vi "PicoScope4000GetBlock.vi"(0 "error in":errorcluster, 2 "handle in":i16, 3 "Acquisition Settings":T3 {"Down Sample Ratio" min=1 step=1}) -> (4 "overflow":i16, 6 "error out":errorcluster, 7 "handle out":i16, 9 "Buffers (Max or non-aggregated)":T1, 10 "Min Buffers":T2)   [LabVIEW 2009]
doc: "This VI collects a block of data from the oscilloscope. This can be called in a loop in order to continually collect blocks of data. The oscilloscope should first be set up by using PicoScope4000Settings.vi. The VI outputs data arrays in two clusters (max and min). If not using aggregation, 'Min Buffers' is not used."
uses:
  ps4000.dll
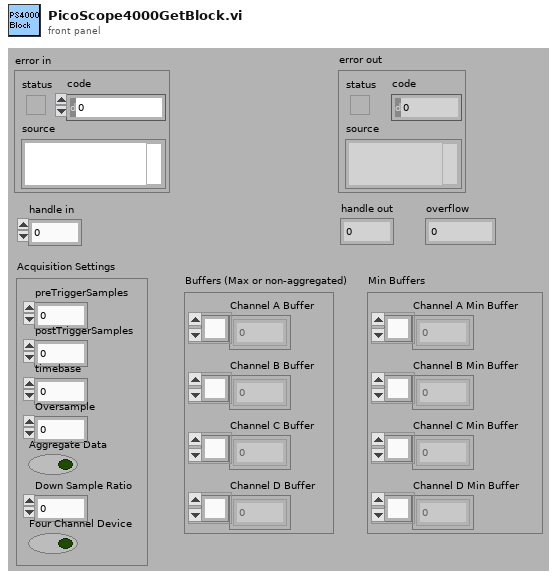
[diagram p1: front panel]
types:
  T1 = cluster{"Channel D Buffer":i16[], "Channel C Buffer":i16[], "Channel B Buffer":i16[], "Channel A Buffer":i16[]}
  T2 = cluster{"Channel A Min Buffer":i16[], "Channel B Min Buffer":i16[], "Channel C Min Buffer":i16[], "Channel D Min Buffer":i16[]}
  T3 = cluster{"preTriggerSamples":i32, "postTriggerSamples":i32, "timebase":u32, "Aggregate Data":bool, "Down Sample Ratio":u32, "Four Channel Device":bool, "Oversample":i16}
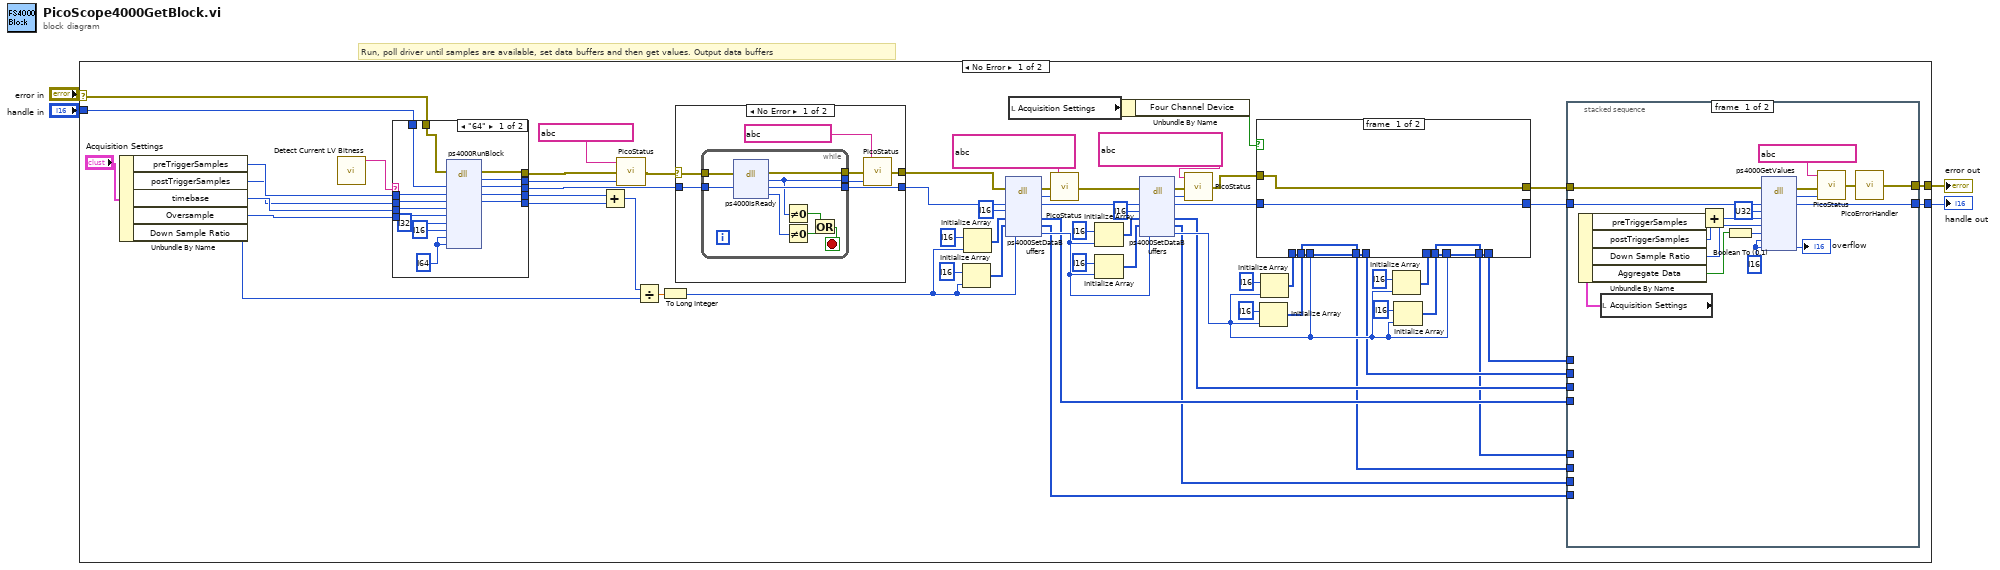
[diagram p0: block diagram]
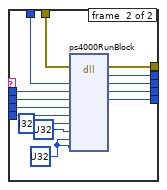
[diagram p2: hidden frame]
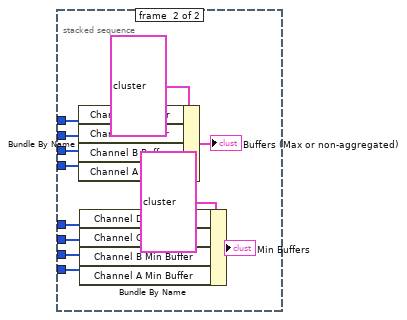
[diagram p3: hidden frame]
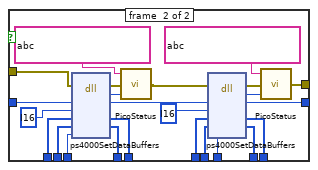
[diagram p5: hidden frame]
diagram:
  # "Run, poll driver until samples are available, set data buffers and then get values. Output data buffers"
  n1 = case shown="No Error" "error in" {
    selector: "error in" -> [w33 w177]
    tunnel: [w34 w177] -> w3
    tunnel: "handle in" -> [w32 w176]
    tunnel: [w31 w176] -> w1
    frame #0 {
      n2 = Unbundle By Name("Acquisition Settings") -> ("preTriggerSamples"=w50:i32, "postTriggerSamples"=w49:i32, "timebase"=w51:u32, "Oversample"=w6:i16, "Down Sample Ratio"=w7:u32)
      n3 = call "Detect Current LV Bitness.vi"() -> ("bitness"=w5:string)  [unwired: 11 in]
      n4 = case shown="\"64\"" w5 {
        tunnel: [w72 w97] -> w69
        tunnel: [w71 w96] -> w64
        tunnel: [w70 w95] -> w63
        tunnel: w51 -> [w79 w94]
        tunnel: w50 -> [w81 w93]
        tunnel: w49 -> [w80 w92]
        tunnel: [w73 w91] -> w46
        tunnel: [w74 w90] -> w45
        tunnel: w33 -> [w83 w89]
        tunnel: w32 -> [w82 w88]
        tunnel: w6 -> [w78 w87]
        frame #0 {
          w75 = i64 ? ("lpReady")
          n5 = dll-call lib="ps4000.dll" fn="ps4000RunBlock" ("ps3000.dll:_ps3000_open_unit@0")(error in=w83, "handle"=w82, "preTriggerSamples"=w81, "postTriggerSamples"=w80, "timebase"=w79, "oversample"=w78, "timeindisposed"=i32 ?, "segmentIndex"=i16 ?, "lpReady"=w75, "pParameter"=w75) -> (error out=w74:errorcluster, "PICO_STATUS"=w73:i32, "handle"=w72:i16, "preTriggerSamples"=w71:i32, "postTriggerSamples"=w70:i32)  [unwired: 8 in, 1 out]
        }
        frame #1 {
          w84 = u32 ? ("lpReady")
          n6 = dll-call lib="ps4000.dll" fn="ps4000RunBlock" ("ps3000.dll:_ps3000_open_unit@0")(error in=w89, "handle"=w88, "preTriggerSamples"=w93, "postTriggerSamples"=w92, "timebase"=w94, "oversample"=w87, "timeindisposed"=i32 ?, "segmentIndex"=u32 ?, "lpReady"=w84, "pParameter"=w84) -> (error out=w90:errorcluster, "PICO_STATUS"=w91:i32, "handle"=w97:i16, "preTriggerSamples"=w96:i32, "postTriggerSamples"=w95:i32)  [unwired: 8 in, 1 out]
        }
      }
      n7 = Add(x=w64, y=w63) -> (x+y=w10:i32)
      n8 = call "PicoStatus.vi"("PICO STATUS"=w46, "error in"=w45, "source"=string ?) -> ("error out"=w44:errorcluster)
      n9 = Divide(x=w10, y=w7) -> (x/y=w9:dbl)
      n10 = To Long Integer(number=w9) -> (32bit integer=w8:i32)
      n11 = case shown="No Error" w44 {
        selector: w44 -> [w132 w144]
        tunnel: w69 -> [w134 w145]
        tunnel: [w133 w145] -> w68
        tunnel: [w131 w144] -> w55
        frame #0 {
          n12 = while {
            tunnel: [w143] -> w133
            tunnel: w134 -> [w142]
            tunnel: [w137] -> w129
            tunnel: w132 -> [w136]
            tunnel: [w135] -> w130
            stop <- w141 stop-if-true
            n13 = dll-call lib="ps4000.dll" fn="ps4000IsReady" ("ps3000.dll:_ps3000_open_unit@0")(error in=w136, "handle"=w142) -> (error out=w135:errorcluster, "status"=w137:i32, "handle"=w143:i16, "ready"=w138:i16)  [unwired: 3 in, 1 out]
            n14 = Not Equal To 0?(x=w137) -> (x != 0?=w139:bool)
            n15 = Not Equal To 0?(x=w138) -> (x != 0?=w140:bool)
            n16 = Or(x=w139, y=w140) -> (x .or. y?=w141:bool)
          }
          n17 = call "PicoStatus.vi"("PICO STATUS"=w129, "error in"=w130, "source"=string ?) -> ("error out"=w131:errorcluster)
        }
        frame #1 {
        }
      }
      n18 = Initialize Array(i16 ? ("element"), w8) -> (w29:i16[])
      n19 = Initialize Array(i16 ? ("element"), w8) -> (w62:i16[])
      n20 = dll-call lib="ps4000.dll" fn="ps4000SetDataBuffers" ("ps3000.dll:_ps3000_open_unit@0")(error in=w55, "handle"=w68, "channel"=i16 ?, "bufferMax"=w62, "bufferMin"=w29, "bufferLth"=w8) -> (error out=w42:errorcluster, "PICO_STATUS"=w43:i32, "handle"=w67:i16, "bufferMax"=w15:i16[], "bufferMin"=w11:i16[], "bufferLth"=w20:i32)  [unwired: 3 in, 1 out]
      n21 = local read "Acquisition Settings"() -> (w48:T3)
      n22 = call "PicoStatus.vi"("PICO STATUS"=w43, "error in"=w42, "source"=string ?) -> ("error out"=w41:errorcluster)
      n23 = Initialize Array(i16 ? ("element"), w20) -> (w59:i16[])
      n24 = Initialize Array(i16 ? ("element"), w20) -> (w27:i16[])
      n25 = Unbundle By Name(w48) -> ("Four Channel Device"=w47:bool)
      n26 = dll-call lib="ps4000.dll" fn="ps4000SetDataBuffers" ("ps3000.dll:_ps3000_open_unit@0")(error in=w41, "handle"=w67, "channel"=i16 ?, "bufferMax"=w59, "bufferMin"=w27, "bufferLth"=w20) -> (error out=w39:errorcluster, "PICO_STATUS"=w40:i32, "handle"=w66:i16, "bufferMax"=w16:i16[], "bufferMin"=w12:i16[], "bufferLth"=w19:i32)  [unwired: 3 in, 1 out]
      n27 = call "PicoStatus.vi"("PICO STATUS"=w40, "error in"=w39, "source"=string ?) -> ("error out"=w38:errorcluster)
      n28 = Initialize Array(i16 ? ("element"), w19) -> (w24:i16[])
      n29 = Initialize Array(i16 ? ("element"), w19) -> (w58:i16[])
      n30 = Initialize Array(i16 ? ("element"), w19) -> (w57:i16[])
      n31 = Initialize Array(i16 ? ("element"), w19) -> (w21:i16[])
      n32 = case shown="True" w47 {
        tunnel: w66 -> [w149 w175]
        tunnel: [w149 w173] -> w65
        tunnel: w58 -> [w151 w172]
        tunnel: w57 -> [w150 w171]
        tunnel: [w150 w170] -> w18
        tunnel: [w151 w169] -> w17
        tunnel: w38 -> [w148 w166]
        tunnel: [w148 w160] -> w53
        tunnel: w24 -> [w147 w157]
        tunnel: w21 -> [w146 w156]
        tunnel: [w146 w155] -> w14
        tunnel: [w147 w154] -> w13
        tunnel: w19 -> [_ w153]
        tunnel: w19 -> [_ w152]
        frame #0 {
        }
        frame #1 {
          n33 = dll-call lib="ps4000.dll" fn="ps4000SetDataBuffers" ("ps3000.dll:_ps3000_open_unit@0")(error in=w166, "handle"=w175, "channel"=i16 ?, "bufferMax"=w172, "bufferMin"=w157, "bufferLth"=w153) -> (error out=w164:errorcluster, "PICO_STATUS"=w165:i32, "handle"=w174:i16, "bufferMax"=w169:i16[], "bufferMin"=w154:i16[])  [unwired: 4 in, 1 out]
          n34 = call "PicoStatus.vi"("PICO STATUS"=w165, "error in"=w164, "source"=string ?) -> ("error out"=w163:errorcluster)
          n35 = dll-call lib="ps4000.dll" fn="ps4000SetDataBuffers" ("ps3000.dll:_ps3000_open_unit@0")(error in=w163, "handle"=w174, "channel"=i16 ?, "bufferMax"=w171, "bufferMin"=w156, "bufferLth"=w152) -> (error out=w161:errorcluster, "PICO_STATUS"=w162:i32, "handle"=w173:i16, "bufferMax"=w170:i16[], "bufferMin"=w155:i16[])  [unwired: 4 in, 1 out]
          n36 = call "PicoStatus.vi"("PICO STATUS"=w162, "error in"=w161, "source"=string ?) -> ("error out"=w160:errorcluster)
        }
      }
      n37 = stacked-sequence {
        tunnel: w65 -> [w115 _]
        tunnel: w53 -> [w112 _]
        tunnel: [w107 _] -> w34
        tunnel: [w106 _] -> w31
        tunnel: w18 -> [_ w125]
        tunnel: w17 -> [_ w124]
        tunnel: w16 -> [_ w123]
        tunnel: w15 -> [_ w122]
        tunnel: w14 -> [_ w119]
        tunnel: w13 -> [_ w118]
        tunnel: w12 -> [_ w117]
        tunnel: w11 -> [_ w116]
        frame #0 {
          w113 = i16 ? ("overflow")
          n38 = local read "Acquisition Settings"() -> (w104:T3)
          n39 = Unbundle By Name(w104) -> ("preTriggerSamples"=w99:i32, "postTriggerSamples"=w100:i32, "Down Sample Ratio"=w103:u32, "Aggregate Data"=w101:bool)
          n40 = Add(x=w99, y=w100) -> (x+y=w98:i32)
          n41 = Boolean To (0,1)(Boolean=w101) -> (0, 1=w102:i16)
          n42 = dll-call lib="ps4000.dll" fn="ps4000GetValues" ("ps3000.dll:_ps3000_open_unit@0")(error in=w112, "handle"=w115, "startIndex"=u32 ?, "noOfSamples"=w98, "downSampleRatio"=w103, "downSampleRatioMode"=w102, "segmentIndex"=w113, "overflow"=w113) -> (error out=w110:errorcluster, "PICO_STATUS"=w111:i32, "handle"=w106:i16, "overflow"=→"overflow":i16)  [unwired: 7 in, 1 out]
          n43 = call "PicoStatus.vi"("PICO STATUS"=w111, "error in"=w110, "source"=string ?) -> ("error out"=w108:errorcluster)
          n44 = call "PicoErrorHandler.vi"("error in"=w108) -> ("error out"=w107:errorcluster)
        }
        frame #1 {
          n45 = Bundle By Name(cluster=T1 ? ("Buffers (Max or non-aggregated)"), "Channel D Buffer"=w125, "Channel C Buffer"=w124, "Channel B Buffer"=w123, "Channel A Buffer"=w122) -> (→"Buffers (Max or non-aggregated)":T1)
          n46 = Bundle By Name(cluster=T2 ? ("Min Buffers"), "Channel D Min Buffer"=w119, "Channel C Min Buffer"=w118, "Channel B Min Buffer"=w117, "Channel A Min Buffer"=w116) -> (→"Min Buffers":T2)
        }
      }
    }
    frame #1 {
    }
  }
  "error out" <- w3
  "handle out" <- w1
